vi "ITCMonitor.vi"   [LabVIEW 2015]
uses:
  Instrument_Setup.vi
  Global/Global Variables/Data_Display_global.vi
types:
  T1 = typedef "ITCIO.ctl" = cluster{"Address":T2, "Version":T3, "Ch 1 dec places":i16, "Ch 2 dec places":i16, "Ch 3 dec places":i16, "Ch1 Name":string, "Ch2 Name":string, "Ch3 Name":string}
  T2 = typedef "OxfordAddress.ctl" = cluster{"Com Port":i32, "ISOBUS Address":i32, "GPIB Address":i16, "Communication":enum16{"RS232", "ISOBUS", "GPIB", "Gateway"}}
  T3 = typedef "ITCVersion.ctl" = enum16{"ITC502", "ITC503", "ITC601"}
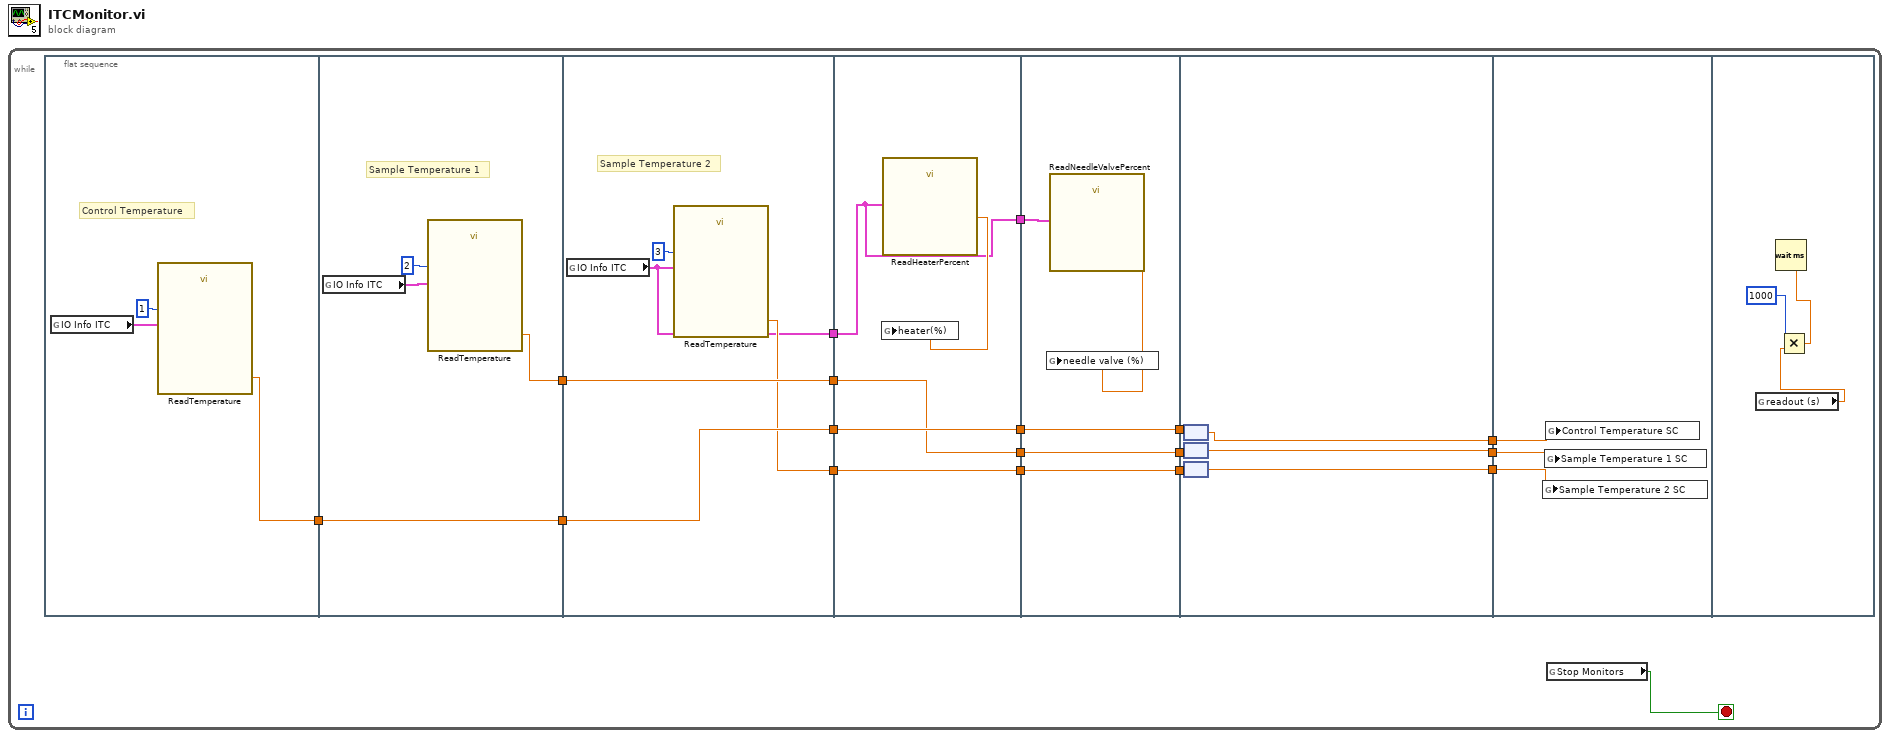
[diagram p0: block diagram]
diagram:
  n1 = while {
    stop <- w9 stop-if-true
    n2 = flat-sequence {
      tunnel: [w19] -> w18
      tunnel: w18 -> [w23]
      tunnel: [w23] -> w17
      tunnel: [w22] -> w16
      tunnel: w17 -> [w29]
      tunnel: w16 -> [w28]
      tunnel: [w29] -> w15
      tunnel: [w28] -> w14
      tunnel: [w27] -> w13
      tunnel: [w26] -> w2
      tunnel: w15 -> [w35]
      tunnel: w14 -> [w34]
      tunnel: w13 -> [w33]
      tunnel: [w35] -> w8
      tunnel: [w34] -> w6
      tunnel: [w33] -> w4
      tunnel: w2 -> [w31]
      tunnel: [w31] -> w1
      tunnel: w8 -> [w40]
      tunnel: [w40] -> w7
      tunnel: w6 -> [w39]
      tunnel: [w39] -> w5
      tunnel: w4 -> [w38]
      tunnel: [w38] -> w3
      tunnel: w1 -> [w36]
      tunnel: w7 -> [w44]
      tunnel: w5 -> [w45]
      tunnel: w3 -> [w46]
      tunnel: [w41] -> w12
      tunnel: [w42] -> w11
      tunnel: [w43] -> w10
      tunnel: w12 -> [w49]
      tunnel: w11 -> [w48]
      tunnel: w10 -> [w47]
      frame #0 {
        # "Control Temperature"
        n3 = global read "Instrument_Setup.vi" "IO Info ITC"() -> (w20:T1)
        n4 = call "ReadTemperature.vi"("Channel"=i16 1, "IO Info"=w20) -> ("Temperature"=w19:dbl[unit])  [unwired: 3 in, 2 out]
      }
      frame #1 {
        # "Sample Temperature 1"
        n5 = global read "Instrument_Setup.vi" "IO Info ITC"() -> (w24:T1)
        n6 = call "ReadTemperature.vi"("Channel"=i16 2, "IO Info"=w24) -> ("Temperature"=w22:dbl[unit])  [unwired: 3 in, 2 out]
      }
      frame #2 {
        # "Sample Temperature 2"
        n7 = global read "Instrument_Setup.vi" "IO Info ITC"() -> (w26:T1)
        n8 = call "ReadTemperature.vi"("Channel"=i16 3, "IO Info"=w26) -> ("Temperature"=w27:dbl[unit])  [unwired: 3 in, 2 out]
      }
      frame #3 {
        n9 = call "ReadHeaterPercent.vi"("ITC IO Info"=w31) -> ("Actual heater  %"=w32:dbl)  [unwired: 1 in, 1 out]
        n10 = global write "Data_Display_global.vi" "heater(%)"(w32) -> ()
      }
      frame #4 {
        n11 = call "ReadNeedleValvePercent.vi"("IO Info"=w36) -> ("Actual Needle Valve  %"=w37:dbl)  [unwired: 1 in, 1 out]
        n12 = global write "Data_Display_global.vi" "needle valve (%)"(w37) -> ()
      }
      frame #5 {
        n13 = node(w44) -> (w43:dbl)
        n14 = node(w45) -> (w42:dbl)
        n15 = node(w46) -> (w41:dbl)
      }
      frame #6 {
        n16 = global write "Data_Display_global.vi" "Sample Temperature 2 SC"(w49) -> ()
        n17 = global write "Data_Display_global.vi" "Sample Temperature 1 SC"(w48) -> ()
        n18 = global write "Data_Display_global.vi" "Control Temperature SC"(w47) -> ()
      }
      frame #7 {
        n19 = global read "Instrument_Setup.vi" "readout (s)"() -> (w50:dbl)
        n20 = Multiply(x=1000, y=w50) -> (x*y=w51:dbl)
        n21 = Wait (ms)(milliseconds to wait=w51) -> ()  [unwired: 1 out]
      }
    }
    n22 = global read "Data_Display_global.vi" "Stop Monitors"() -> (w9:bool)
  }
